vi "Hz to RPM.vi"(9 "Scale Mod":dbl=1.0, 11 "Hz":dbl) -> (3 "RPM":dbl)   [LabVIEW 2020]
doc: "Converts frequency from Hz to RPM. By defeault, setting is configured for standard multiplication of 60. This can be adjusted by Scale Factor control."
panel:
  # "Frequency Conversion (Hz to RPM)"
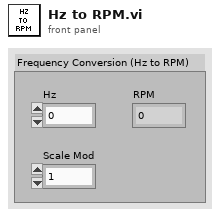
[diagram p1: front panel]
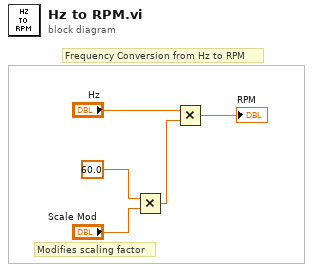
[diagram p0: block diagram]
diagram:
  # "Frequency Conversion from Hz to RPM"
  # "Modifies scaling factor"
  n1 = Multiply(x=60.0 ("y"), y="Scale Mod") -> (x*y=w1:dbl)
  n2 = Multiply(x="Hz", y=w1) -> (x*y=→"RPM":dbl)
